vi "exec.vi"(8 "error in (no error)":errorcluster, 10 "context":refnum<class "IContextThisComponent.lvclass">, 11 "Start in":refnum<class "start.lvclass">) -> (0 "error out":errorcluster, 2 "context 2":refnum<class "IContextThisComponent.lvclass">, 3 "Start out":refnum<class "start.lvclass">)   [LabVIEW 2016, in "Commands.lvlib" / "start.lvclass"]
uses:
  start.lvclass
  IContextThisComponent/IContextThisComponent.lvclass
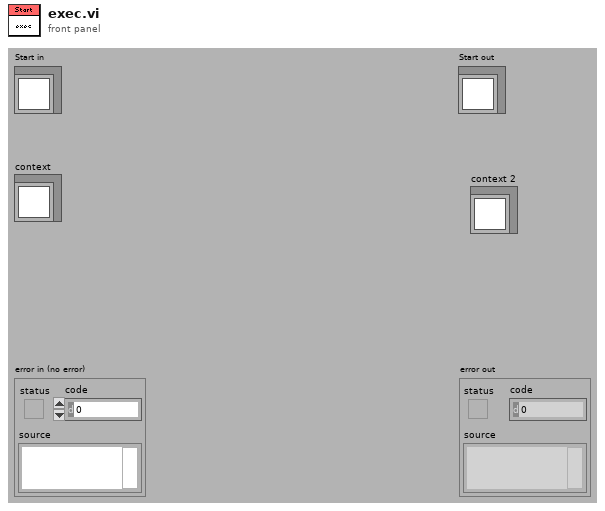
[diagram p1: front panel]
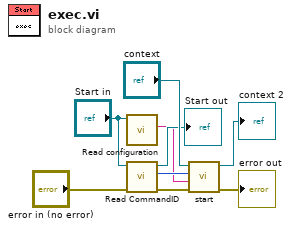
[diagram p0: block diagram]
diagram:
  n1 = call-dynamic "Read configuration.vi"("Start in"="Start in") -> ("configuration"=w1:string)  [unwired: 8 in, 2 out]
  n2 = call-dynamic "Read CommandID.vi"("error in (no error)"="error in (no error)", "Command in"="Start in") -> ("error out"=w5:errorcluster, "CommandID"=w4:i32, "Command out"=→"Start out":refnum<class "start.lvclass">)  [unwired: 7 in]
  n3 = call-dynamic "start.vi"("error in (no error)"=w5, "Configuration"=w1, "CommandID"=w4, "IContextThisComponent in"="context") -> ("error out"=→"error out":errorcluster, "IContextThisComponent out"=→"context 2":refnum<class "IContextThisComponent.lvclass">)  [unwired: 6 in]
